vi "Write Results.lvclass.vi"(8 "error in (no error)":errorcluster, 10 "Results.lvclass":refnum<class "Results.lvclass">, 11 "Send Results Object in":refnum<class "Send Results Object.lvclass">) -> (0 "error out":errorcluster, 3 "Send Results Object out":refnum<class "Send Results Object.lvclass">)   [LabVIEW 2017, in "Controller Actor.lvlib" / "Send Results Object.lvclass"]
uses:
  Send Results Object.lvclass
  Results/Results.lvclass
  Send Results Object.lvclass/Send Results Object.ctl
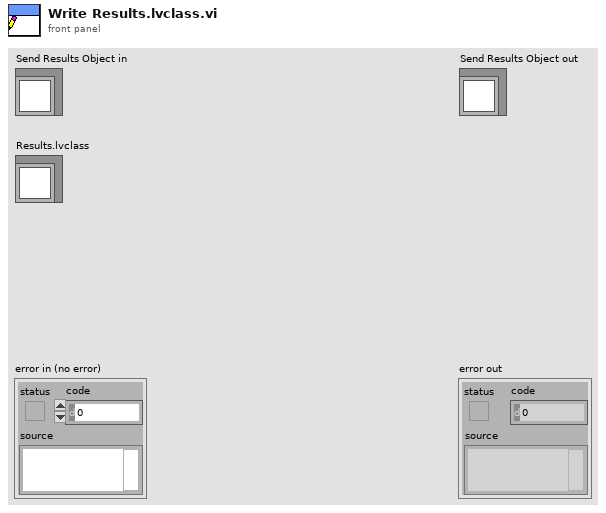
[diagram p1: front panel]
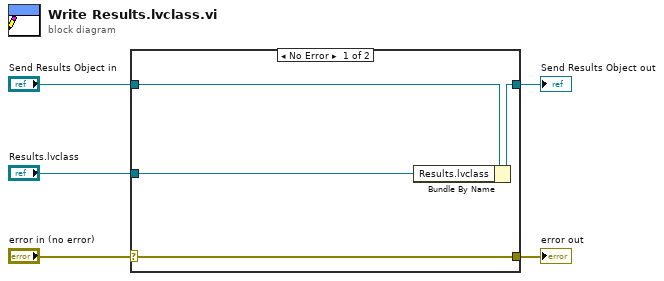
[diagram p0: block diagram]
diagram:
  n1 = case shown="No Error" "error in (no error)" {
    selector: "error in (no error)" -> [w9 w10]
    tunnel: [w9 w10] -> w4
    tunnel: [w7 w11] -> w2
    tunnel: "Send Results Object in" -> [w8 w11]
    tunnel: "Results.lvclass" -> [w6 _]
    frame No Error {
      n2 = Bundle By Name(cluster=w8, "Results.lvclass"=w6) -> (w7:refnum<class "Send Results Object.lvclass">)
    }
    frame Error {
    }
  }
  "error out" <- w4
  "Send Results Object out" <- w2
